vi "Configure FPGA.vi"(8 "error in":errorcluster) -> (0 "error out":errorcluster, 3 "Refnum out":refnum<k20>)   [LabVIEW 2014]
uses:
  <vilib>/FPGAPlugInAG/cRIO-9073/niLvFpga_Open_cRIO-9073.vi
  <vilib>/rvi/interface/common/dynamic/niFpgaDynamicAddResources.vi
  <vilib>/FPGAPlugInAG/Dynamic/niLvFpga_Reset_Dynamic.vi
  <vilib>/Utility/error.llb/Error Cluster From Error Code.vi
  <vilib>/rvi/errors/niLvFpgaAdjustHostInterfaceError.vi
  <vilib>/rvi/interface/common/niFpgaWaitOnOcc.vi
  <vilib>/FPGAPlugInAG/Dynamic/niLvFpga_Run_Dynamic.vi
  <vilib>/RVI Host/nirviSupport.llb/nirviErrorClusterFromErrorCode.vi
  <vilib>/rvi/interface/nirviOpenFPGA/nirviOpenFPGA.xnode
  FPGA Bitfiles/CLEDPrac_FPGATargetcRIO-9_FPGAMain_zcRFuQSVCIk.lvbitx
  <vilib>/rvi/interface/nirviMethod/nirviMethod.xnode
  <vilib>/rvi/interface/nirviReadWriteControl/nirviReadWriteControl.xnode
  NiFpgaLv.dll
  <vilib>/rvi/interface/Simulation/niFpgaSimulationCallBeginRW.vi
  <vilib>/FPGAPlugInAG/Dynamic/niLvFpga_ConfigureFifo_Dynamic.vi
  <vilib>/rvi/errors/niLvFpgaMergeErrorWithErrorCode.vi
  <vilib>/rvi/interface/nirviMethod/StockFPGA_InlinedMethodWaitForSingleIRQ.vi
  <vilib>/FPGAPlugInAG/Dynamic/niLvFpga_WaitOnIrq_Dynamic.vi
  <vilib>/FPGAPlugInAG/Dynamic/niLvFpga_AcknowledgeIrq_Dynamic.vi
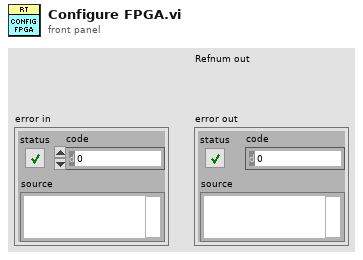
[diagram p1: front panel]
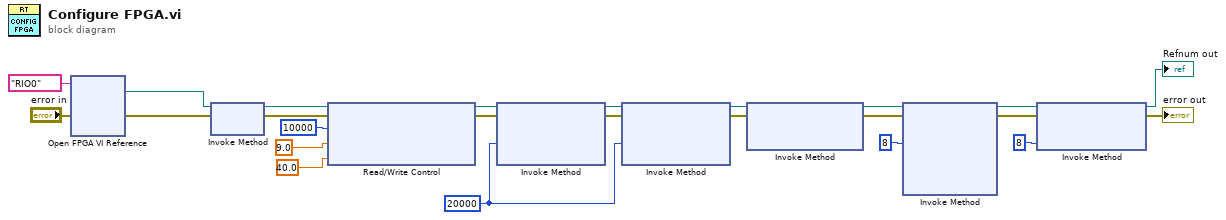
[diagram p0: block diagram]
diagram:
  w15 = u32 20000 ("Requested Depth")
  n1 = xnode "Open FPGA VI Reference"("error in"="error in", "resource name"=tag "RIO0") -> ("FPGA VI Reference Out"=w3:refnum<k20>, "error out"=w7:errorcluster)
  n2 = xnode "Invoke Method"("FPGA VI Reference In"=w3, "error in"=w7) -> ("FPGA VI Reference Out"=w4:refnum<k20>, "error out"=w6:errorcluster)
  n3 = xnode "Read/Write Control"("FPGA VI Reference In"=w4, "error in"=w6, "Siimulator Time out value"=u32 10000, "pH Threshold"=sgl 9.0, "Temp Threshold"=sgl 40.0) -> ("FPGA VI Reference Out"=w5:refnum<k20>, "error out"=w13:errorcluster)
  n4 = xnode "Invoke Method"("FPGA VI Reference In"=w5, "error in"=w13, "Requested Depth"=w15) -> ("FPGA VI Reference Out"=w11:refnum<k20>, "error out"=w14:errorcluster)  [unwired: 1 out]
  n5 = xnode "Invoke Method"("FPGA VI Reference In"=w11, "error in"=w14, "Requested Depth"=w15) -> ("FPGA VI Reference Out"=w12:refnum<k20>, "error out"=w16:errorcluster)  [unwired: 1 out]
  n6 = xnode "Invoke Method"("FPGA VI Reference In"=w12, "error in"=w16) -> ("FPGA VI Reference Out"=w17:refnum<k20>, "error out"=w18:errorcluster)  [unwired: 1 in]
  n7 = xnode "Invoke Method"("FPGA VI Reference In"=w17, "error in"=w18, "IRQ Number(s)"=8) -> ("FPGA VI Reference Out"=w20:refnum<k20>, "error out"=w21:errorcluster)  [unwired: 1 in, 2 out]
  n8 = xnode "Invoke Method"("FPGA VI Reference In"=w20, "error in"=w21, "IRQ Number(s)"=8) -> ("FPGA VI Reference Out"=→"Refnum out":refnum<k20>, "error out"=→"error out":errorcluster)
